vi "LoadCombo.vi"() -> ()   [LabVIEW 2016]
panel:
  in  "LoadCombo":i32[](array[numeric])
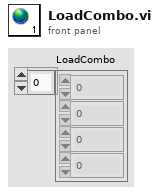
[diagram p1: front panel]
diagram:
